vi "数组至excel行.vi"(11 "数组":string[](array[string])) -> (3 "字符串":string)   [LabVIEW 2017]
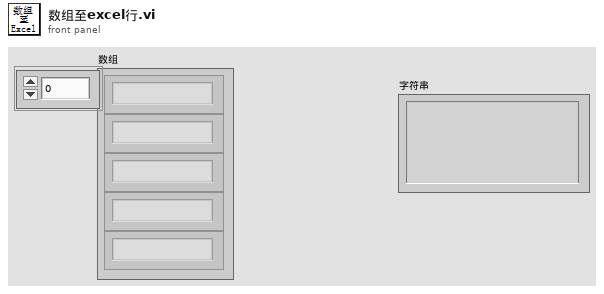
[diagram p1: front panel]
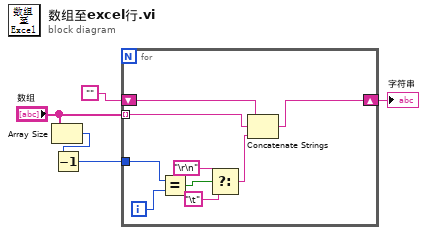
[diagram p0: block diagram]
diagram:
  n1 = Array Size(array="数组") -> (size(s)=w4:i32)
  n2 = Decrement(x=w4) -> (x-1=w3:i32)
  n3 = for {
    tunnel: "数组" -> [w14] mode=indexing
    tunnel: w3 -> [w12]
    shift-right: [w7] -> w1
    shift-left: "" -> [w6]
    i -> [w13]
    n4 = Equal?(x=w12, y=w13) -> (x = y?=w11:bool)
    n5 = Select(t="\r\n", s=w11, f="\t") -> (s? t:f=w8:string)
    n6 = Concatenate Strings(w6, w14, w8) -> (w7:string)
  }
  "字符串" <- w1
